vi "Audio Playback Example (LINX).vi"() -> ()   [LabVIEW 2020]
doc: "Simple example of audio device playback of a file decoded with G-Audio."
uses:
  Controls/Audio Device Config.ctl
  Controls/Audio Device Format.ctl
  8289e2ef-86ba-4438-8a42-485f00fd8c95.vi
  9545a255-db38-479b-bcdc-619f4ee8d9ed.vi
  Private/Get Basic Audio File Info.vi
  Private/Result To Error.vi
  8289e2ef-86ba-4438-8a42-485f00fd8c95.vi/779dfdfd-1b42-4cf4-8001-66d3dd167625.vi
  8289e2ef-86ba-4438-8a42-485f00fd8c95.vi/55d550d4-9624-414e-aebd-6e02b5081896.vi
  Private/Audio File Refnum To Value.vi
  9545a255-db38-479b-bcdc-619f4ee8d9ed.vi/4dfb5711-8d81-45a3-b3db-a84d40650863.vi
  9545a255-db38-479b-bcdc-619f4ee8d9ed.vi/c8869513-30c6-44f2-a2d3-73232fe63870.vi
  Private/Audio Device Refnum To Value.vi
  8289e2ef-86ba-4438-8a42-485f00fd8c95.vi/55d550d4-9624-414e-aebd-6e02b5081896.vi/4b7b629c-2e91-4160-9820-a26af8f6e677.vi
  9545a255-db38-479b-bcdc-619f4ee8d9ed.vi/4dfb5711-8d81-45a3-b3db-a84d40650863.vi/4b7b629c-2e91-4160-9820-a26af8f6e677.vi
  9545a255-db38-479b-bcdc-619f4ee8d9ed.vi/c8869513-30c6-44f2-a2d3-73232fe63870.vi/4b7b629c-2e91-4160-9820-a26af8f6e677.vi
  Audio Files/Polymorphic VIs/Get Audio File Info (Path).vi
  Audio Files/Polymorphic VIs/Open Audio File Read (Path).vi
  <vilib>/Utility/Data Type/Get Numeric Information.vi
  <vilib>/Utility/error.llb/Error Cluster From Error Code.vi
  G-Audio.lvlib
panel:
  out "Waveform":waveform(i16)[](graph)
  in  "Now Playing:":path=path "/home/pi/music.mp3"
  out "Duration":string
  out "Sample Length":u64
  out "Audio Info":T1
  out "error out":errorcluster
  in  "Stop":bool
  # "Instructions:\n1. Ensure G-Audio has been installed on the LINX target. See block diagram for detailed instructions.\n2. Enter the path to an audio file on the LINX target (e.g. /home/pi/music.mp3).\n3. Run the VI.\n4. The VI will stop when the file has finished playing, or when the Stop button is pressed."
  # "G"
  # "-Audio"
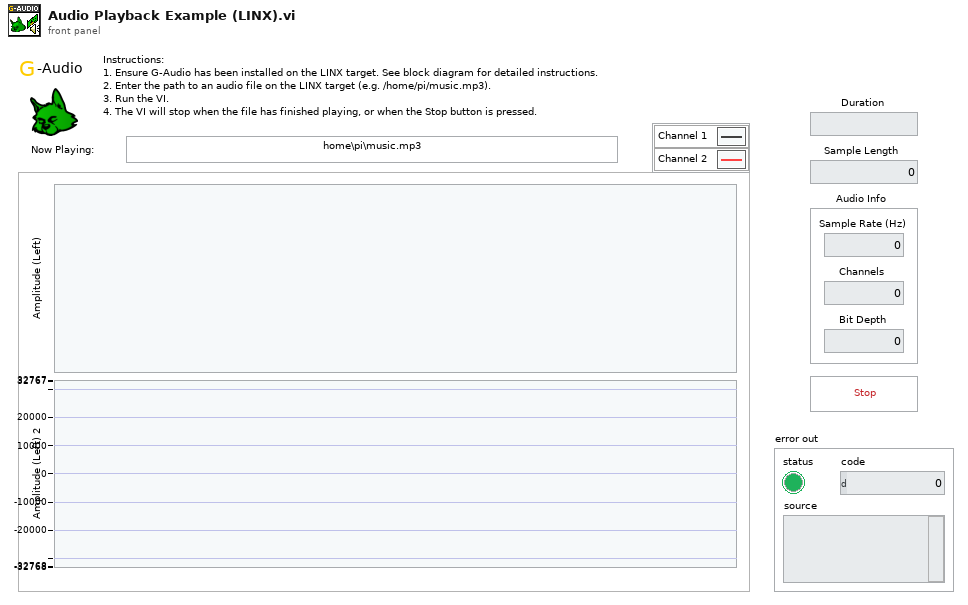
[diagram p1: front panel]
types:
  T1 = cluster{"Sample Rate (Hz)":u32, "Channels":u32, "Bit Depth":u32}
  T2 = typedef "G-Audio.lvlib/Audio Device Config.ctl" = cluster{"Sample Rate (Hz)":u32, "Channels":u32, "Format":T3}
  T3 = typedef "G-Audio.lvlib/Audio Device Format.ctl" = enum16{"Native", "U8", "I16", "I32", "SGL"}
  T4 = typedef "G-Audio.lvlib/Audio File Info.ctl" = cluster{"Sample Rate (Hz)":u32, "Channels":u32, "Bit Depth":u32}
  T5 = typedef "G-Audio.lvlib/Audio File Refnum.ctl" = refnum<file>
  T6 = typedef "G-Audio.lvlib/Audio Device Refnum.ctl" = refnum<file>
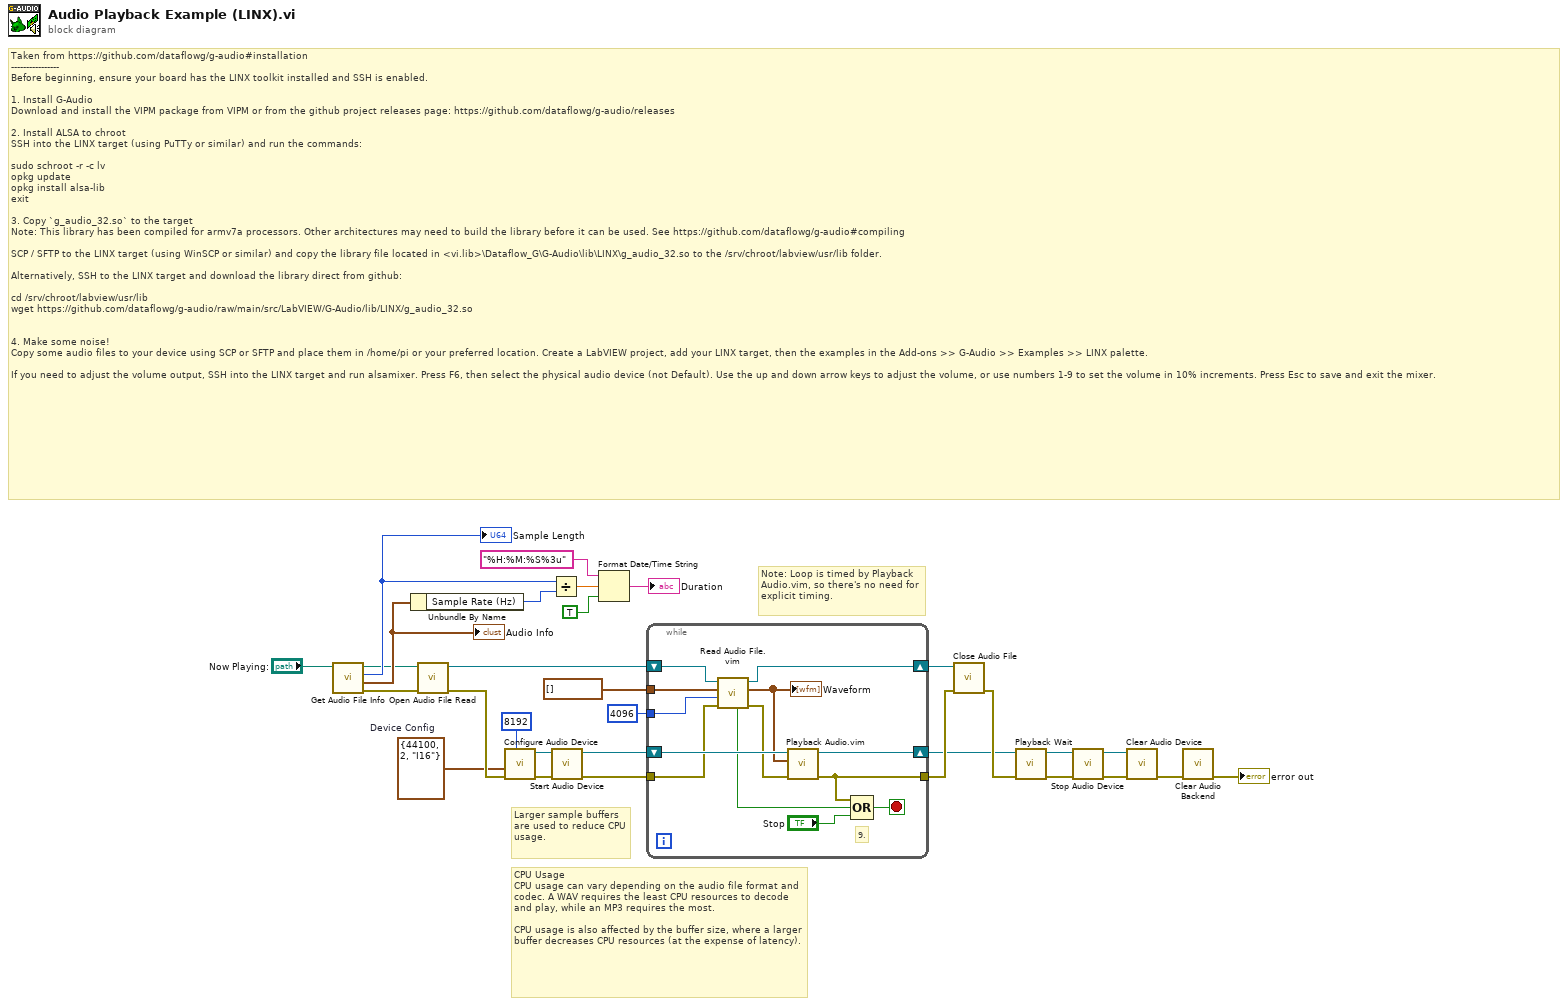
[diagram p0: block diagram]
diagram:
  w6 = T2 {"Sample Rate (Hz)"=44100, "Channels"=2, "Format"=enum."I16"}  # Device Config
  # "Taken from https://github.com/dataflowg/g-audio#installation \n----------------\nBefore beginning, ensure your board has the LINX toolkit installed and SSH is enabled.\n\n1. Install G-Audio\nDownload and install the VIPM package from VIPM or from the github project releases page: https://github.com/dataflowg/g-audio/releases \n\n2. Install ALSA to chroot\nSSH into the LINX target (using PuTTy or similar) and run the commands:\n\nsudo schroot -r -c lv\nopkg update\nopkg install alsa-lib\nexit\n\n3. Copy `g_audio_32.so` to the target\nNote: This library has been compiled for armv7a processors. Other architectures may need to build the library before it can be used. See https://github.com/dataflowg/g-audio#compiling\n\nSCP / SFTP to the LINX target (using WinSCP or similar) and copy the library file located in <vi.lib>\\Dataflow_G\\G-Audio\\lib\\LINX\\g_audio_32.so to the /srv/chroot/labview/usr/lib folder.\n\nAlternatively, SSH to the LINX target and download the library direct from github:\n\ncd /srv/chroot/labview/usr/lib\nwget https://github.com/dataflowg/g-audio/raw/main/src/LabVIEW/G-Audio/lib/LINX/g_audio_32.so\n\n\n4. Make some noise!\nCopy some audio files to your device using SCP or SFTP and place them in /home/pi or your preferred location. Create a LabVIEW project, add your LINX target, then the examples in the Add-ons >> G-Audio >> Examples >> LINX palette.\n\nIf you need to adjust the volume output, SSH into the LINX target and run alsamixer. Press F6, then select the physical audio device (not Default). Use the up and down arrow keys to adjust the volume, or use numbers 1-9 to set the volume in 10% increments. Press Esc to save and exit the mixer."
  # "CPU Usage\nCPU usage can vary depending on the audio file format and codec. A WAV requires the least CPU resources to decode and play, while an MP3 requires the most.\n\nCPU usage is also affected by the buffer size, where a larger buffer decreases CPU resources (at the expense of latency)."
  # "Larger sample buffers are used to reduce CPU usage."
  # "Note: Loop is timed by Playback Audio.vim, so there's no need for explicit timing."
  n1 = call-poly "Get Audio File Info.vi"("Path In"="Now Playing:") -> ("error out"=w29:errorcluster, "Audio File Info"=w18:T4, "PCM Frame Length"=w19:u64, "Path Out"=w3:path)  [unwired: 6 in, 1 out]
  "Audio Info" <- w18
  "Sample Length" <- w19
  n2 = Unbundle By Name(w18) -> ("Sample Rate (Hz)"=w17:u32)
  n3 = call-poly "Open Audio File Read.vi"("error in (no error)"=w29, "Path"=w3) -> ("error out"=w7:errorcluster, "Audio File Refnum"=w20:T5)  [unwired: 8 in]
  n4 = call "Configure Audio Device.vi"("Buffer Size (4096)"=8192 ("number of samples/ch"), "error in (no error)"=w7, "Device Config"=w6) -> ("error out"=w13:errorcluster, "Audio Device Refnum"=w12:T6)  [unwired: 5 in, 2 out]
  n5 = Divide(x=w19, y=w17) -> (x/y=w16:dbl)
  n6 = call "Start Audio Device.vi"("error in (no error)"=w13, "Audio Device Refnum In"=w12) -> ("error out"=w22:errorcluster, "Audio Device Refnum Out"=w23:T6)  [unwired: 8 in]
  n7 = Format Date/Time String(time format string (%c)="%H:%M:%S%3u", seconds (now)=w16, UTC format=TRUE) -> (date/time string=→"Duration":string)
  n8 = while {
    shift-right: [w41] -> w28
    shift-left: w20 -> [w43]
    shift-right: [w40] -> w9
    shift-left: w23 -> [w42]
    tunnel: w22 -> [w39]
    tunnel: [w34] -> w26
    tunnel: u64 4096 ("number of samples/ch") -> [w33]
    tunnel: waveform(i16)[] [] -> [w32]
    stop <- w36 stop-if-true
    # "9."
    n9 = call "Read Audio File.vim"("error in (no error)"=w39, "Frames To Read"=w33, "Data Format"=w32, "Audio File Refnum In"=w43) -> ("error out"=w38:errorcluster, "Audio Data"=w31:waveform(i16)[], "Audio File Refnum Out"=w41:T5, "End of File?"=w37:bool)  [unwired: 3 in, 1 out]
    "Waveform" <- w31
    n10 = call "Playback Audio.vim"("error in (no error)"=w38, "Audio Data"=w31, "Audio Device Refnum In"=w42) -> ("error out"=w34:errorcluster, "Audio Device Refnum Out"=w40:T6)  [unwired: 7 in]
    n11 = Compound Arithmetic op=OR(w34, w37, "Stop") -> (w36:bool)
  }
  n12 = call "Close Audio File.vi"("error in (no error)"=w26, "Audio File Refnum In"=w28) -> ("error out"=w25:errorcluster)  [unwired: 9 in]
  n13 = call "Playback Wait.vi"("error in (no error)"=w25, "Audio Device Refnum In"=w9) -> ("error out"=w10:errorcluster, "Audio Device Refnum Out"=w8:T6)  [unwired: 8 in]
  n14 = call "Stop Audio Device.vi"("error in (no error)"=w10, "Audio Device Refnum In"=w8) -> ("error out"=w24:errorcluster, "Audio Device Refnum Out"=w27:T6)  [unwired: 8 in]
  n15 = call "Clear Audio Device.vi"("error in (no error)"=w24, "Audio Device Refnum In"=w27) -> ("error out"=w21:errorcluster)  [unwired: 9 in]
  n16 = call "Clear Audio Backend.vi"("error in (no error)"=w21) -> ("error out"=→"error out":errorcluster)  [unwired: 10 in]
